vi "MeasureBaselineCurrents.vi"   [LabVIEW 2020]
doc: "Measures and reports the baseline PDH currents during a systems check."
uses:
  robotconstants.vi
  driverdata.vi
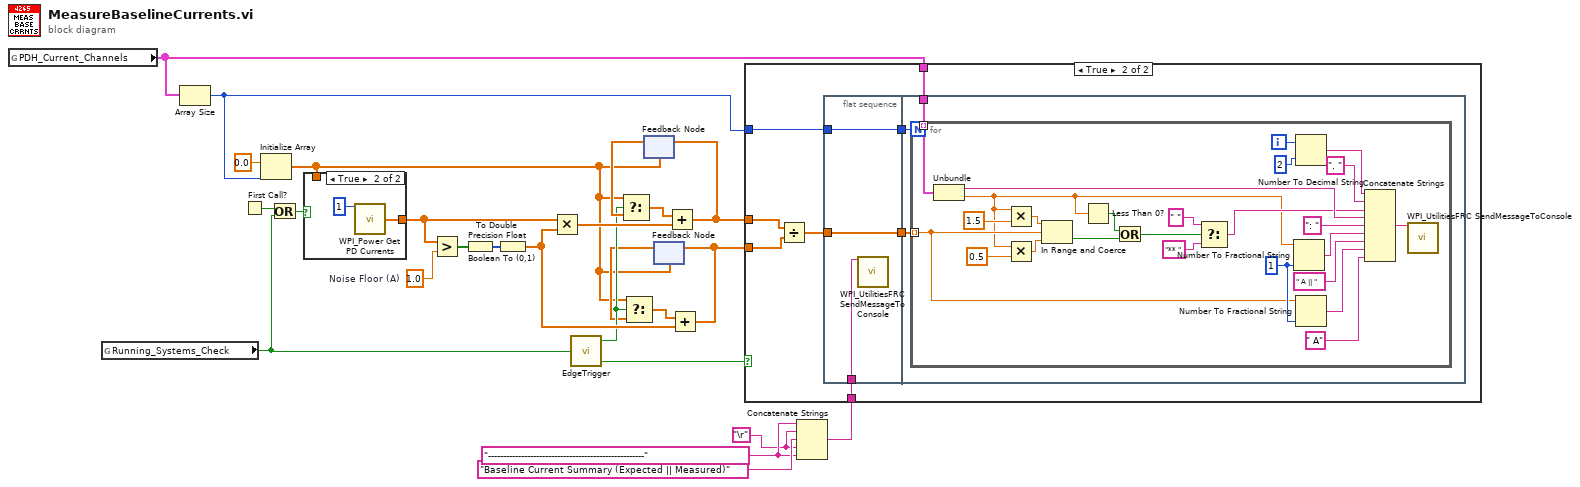
[diagram p0: block diagram]
diagram:
  w2 = "----------------------------------------------------" ("string")
  w1 = "\r"
  w22 = 1.0  # Noise Floor (A)
  n1 = global read "robotconstants.vi" "PDH_Current_Channels"() -> (w3:cluster{string, dbl}[])
  n2 = global read "driverdata.vi" "Running_Systems_Check"() -> (w5:bool)
  n3 = Array Size(array=w3) -> (size(s)=w4:i32)
  n4 = First Call?() -> (First Call?: T/F=w9:bool)
  n5 = Initialize Array(0.0 ("element"), w4) -> (w8:dbl[])
  n6 = Or(x=w9, y=w5) -> (x .or. y?=w10:bool)
  n7 = case shown="True" w10 {
    tunnel: [w26 w27] -> w19
    tunnel: w8 -> [w26 _]
    frame False {
    }
    frame True {
      n8 = call <vilib>:"WPI_Power Get PD Currents.vi"("Power Distribution (def)"=u8 1) -> ("all currents (A)"=w27:dbl[])  [unwired: 11 in, 3 out]
    }
  }
  n9 = Greater?(x=w19, y=w22) -> (0:w21:bool[])
  n10 = Boolean To (0,1)(Boolean=w21) -> (0, 1=w20:i16[])
  n11 = To Double Precision Float(number=w20) -> (double precision float=w16:dbl[])
  n12 = Multiply(x=w19, y=w16) -> (x*y=w18:dbl[])
  n13 = call "EdgeTrigger.vi"("Input Signal"=w5) -> ("Rising Edge Trigger"=w15:bool, "Falling Edge Trigger"=w11:bool)  [unwired: 1 out]
  n14 = feedback #1(w8) -> (w24:dbl[])
  n15 = Select(t=w8, s=w15, f=w24) -> (s? t:f=w23:dbl[])
  n16 = feedback #2(w8) -> (w14:dbl[])
  n17 = Select(t=w8, s=w15, f=w14) -> (s? t:f=w17:dbl[])
  n18 = Add(x=w23, y=w18) -> (x+y=w13:dbl[])
  n19 = feedback-in #1(w13) -> ()
  n20 = Add(x=w17, y=w16) -> (x+y=w12:dbl[])
  n21 = feedback-in #2(w12) -> ()
  n22 = Concatenate Strings(w2, w1, "Baseline Current Summary (Expected || Measured)" ("Message"), w1, w2) -> (w7:string)
  n23 = case shown="True" w11 {
    tunnel: w13 -> [_ w36]
    tunnel: w12 -> [_ w35]
    tunnel: w4 -> [_ w33]
    tunnel: w7 -> [_ w30]
    tunnel: w3 -> [_ w29]
    frame False {
    }
    frame True {
      n24 = Divide(x=w36, y=w35) -> (x/y=w34:dbl[])
      n25 = flat-sequence {
        tunnel: w33 -> [w38]
        tunnel: w34 -> [w39]
        tunnel: [w39] -> w32
        tunnel: [w38] -> w31
        tunnel: w30 -> [w37]
        tunnel: w32 -> [w42]
        tunnel: w31 -> [w41]
        tunnel: w29 -> [w40]
        frame #0 {
          n26 = call <vilib>:"WPI_UtilitiesFRC SendMessageToConsole.vi"("Message"=w37) -> ()  [unwired: 14 in, 1 out]
        }
        frame #1 {
          n27 = for {
            N: w41 -> [_]
            tunnel: w42 -> [w47] mode=indexing
            tunnel: w40 -> [w60] mode=indexing
            i -> [w51]
            w62 = i16 1 ("precision (6)")
            n28 = Unbundle(w60) -> (w59:string, w46:dbl)
            n29 = Multiply(x=w46, y=1.5) -> (x*y=w58:dbl)
            n30 = Multiply(x=w46, y=0.5) -> (x*y=w57:dbl)
            n31 = In Range and Coerce(upper limit=w58, x=w47, lower limit=w57) -> (In Range?=w45:bool)  [unwired: 1 out]
            n32 = Less Than 0?(x=w46) -> (x < 0?=w43:bool)
            n33 = Or(x=w43, y=w45) -> (x .or. y?=w44:bool)
            n34 = Select(t=" ", s=w44, f="** ") -> (s? t:f=w54:string)
            n35 = Number To Fractional String(number=w46, precision (6)=w62) -> (F-format string=w66:string)  [unwired: 2 in]
            n36 = Number To Decimal String(number=w51, width (-)=i16 2) -> (decimal integer string=w49:string)
            n37 = Number To Fractional String(number=w47, precision (6)=w62) -> (F-format string=w67:string)  [unwired: 2 in]
            n38 = Concatenate Strings(w49, ". " ("string"), w54, w59, ": ", w66, " A || ", w67, " A") -> (w61:string)
            n39 = call <vilib>:"WPI_UtilitiesFRC SendMessageToConsole.vi"("Message"=w61) -> ()  [unwired: 14 in, 1 out]
          }
        }
      }
    }
  }
